vi "test_Max Nr Of Scalar Channels_Basic Deployment.vi"(8 "error in (no error)":errorcluster) -> (0 "error out":errorcluster, 2 "System Definition Information":T1)   [LabVIEW 2019, in "Max Nr of Scalar Channels.lvclass"]
uses:
  Max Nr of Scalar Channels.lvclass
  niveristand-custom-device-testing-tools/VeriStandTestUtilities/SystemDefinitionInformation.ctl
  niveristand-custom-device-testing-tools/VeriStandTestUtilities/TargetInformation.ctl
  niveristand-custom-device-testing-tools/VeriStandTestUtilities/ChassisInformation.ctl
  C:/Dev/niveristand-fpga-addon-custom-device/Source/Tests/FPGA Addon Test Class/FPGA Addon Test Class.lvclass
  C:/Dev/niveristand-custom-device-testing-tools/VeriStandTestCase/VeriStandTestCase.lvclass
  FPGA Addon Test Class/FPGA Addon Test Class.lvclass/FPGA Addon Test Class.ctl
  FPGA Addon Test Class/FPGA Addon Test Class.lvclass
  niveristand-custom-device-testing-tools/VeriStandTestUtilities/VeriStandTestUtilities.lvlib
panel:
  out "TestCase out":refnum<class "Max Nr of Scalar Channels.lvclass">
  in  "TestCase in":refnum<class "Max Nr of Scalar Channels.lvclass">
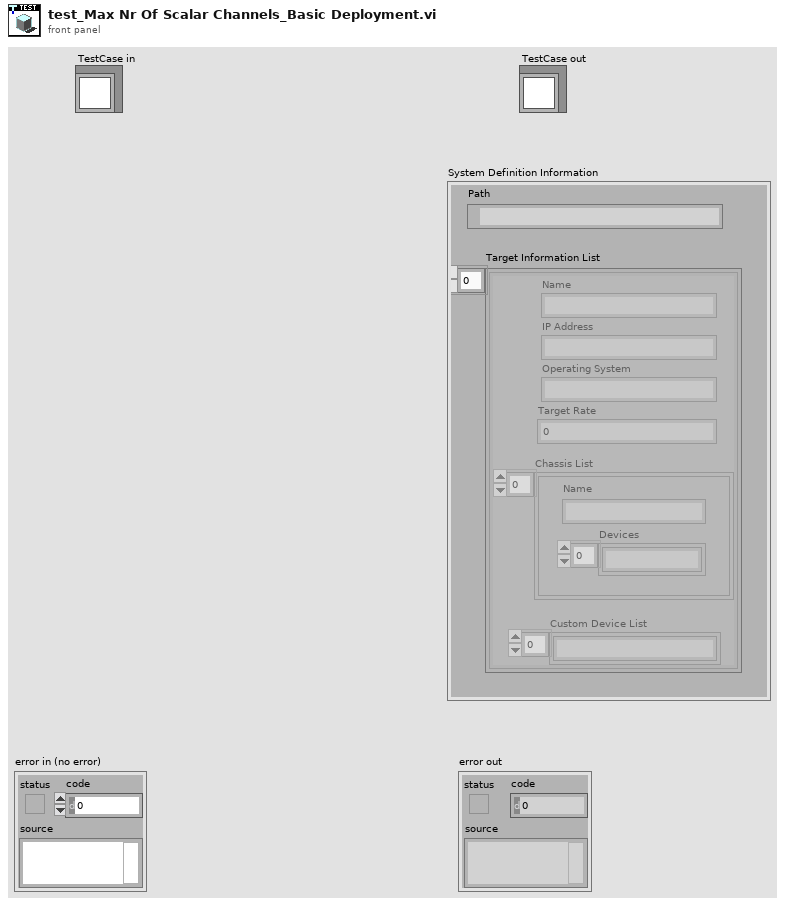
[diagram p1: front panel]
types:
  T1 = typedef "VeriStandTestUtilities.lvlib/SystemDefinitionInformation.ctl" = cluster{"Path":path, "Target Information List":T2[]}
  T2 = typedef "VeriStandTestUtilities.lvlib/TargetInformation.ctl" = cluster{"Name":string, "IP Address":string, "Operating System":string, "Target Rate":dbl, "Chassis List":T3[], "Custom Device List":string[]}
  T3 = typedef "VeriStandTestUtilities.lvlib/ChassisInformation.ctl" = cluster{"Name":string, "Devices":string[]}
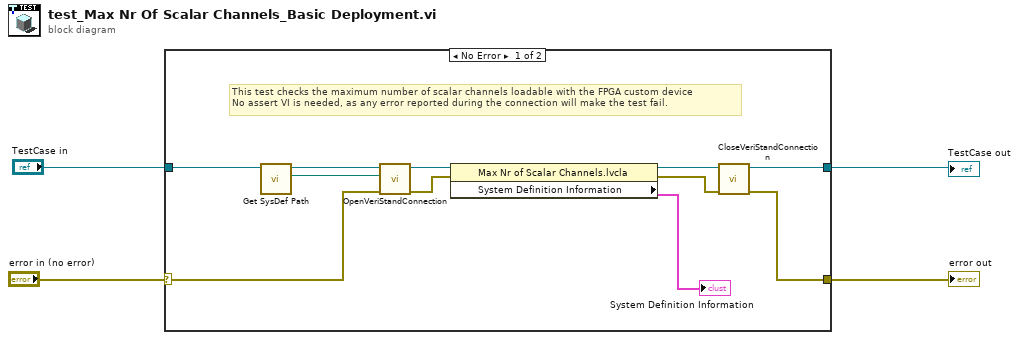
[diagram p0: block diagram]
diagram:
  n1 = case shown="No Error" "error in (no error)" {
    selector: "error in (no error)" -> [w10 w17]
    tunnel: [w9 w17] -> w4
    tunnel: [w11 w16] -> w1
    tunnel: "TestCase in" -> [w7 w16]
    frame No Error {
      # "This test checks the maximum number of scalar channels loadable with the FPGA custom device\nNo assert VI is needed, as any error reported during the connection will make the test fail."
      n2 = call "Get SysDef Path.vi"("Scalar Channels Testing in"=w7) -> ("SysDef Path"=w5:path, "Scalar Channels Testing out"=w6:refnum<class "Max Nr of Scalar Channels.lvclass">)  [unwired: 9 in]
      n3 = call-dynamic "OpenVeriStandConnection.vi"("error in (no error)"=w10, "System Definition File"=w5, "VeriStand Test Case in"=w6) -> ("error out"=w14:errorcluster, "VeriStand Test Case out"=w15:refnum<class "Max Nr of Scalar Channels.lvclass">)  [unwired: 6 in, 1 out]
      n4 = property class="Max Nr of Scalar Channels.lvcla"(reference=w15, error in=w14) -> (reference out=w13:refnum<class "Max Nr of Scalar Channels.lvclass">, error out=w12:errorcluster, "System Definition Information"=→"System Definition Information":T1)
      n5 = call-dynamic "CloseVeriStandConnection.vi"("error in (no error)"=w12, "VeriStand Test Case in"=w13) -> ("error out"=w9:errorcluster, "VeriStand Test Case out"=w11:refnum<class "Max Nr of Scalar Channels.lvclass">)  [unwired: 8 in]
    }
    frame Error {
    }
  }
  "error out" <- w4
  "TestCase out" <- w1
